vi "IMAQ Gerchberg Saxton.vi"(0 "Source":T1, 1 "Target":T1, 2 "Source Phase":T1, 3 "Target Phase":T1, 4 "n_grid":i32=300, 5 "Number of Iteration":i32=50, 6 "size_grid":dbl=0.001776, 7 "forward distance":dbl=0.02, 8 "MF Phase Refnum":refnum<vi>, 9 "FF Refnum":refnum<vi>, 10 "MF Refnum":refnum<vi>, 11 "FF Phase Refnum":refnum<vi>, 12 "lambda":dbl=1.054e-06, 13 "Target Int RMS":refnum<vi>) -> (14 "Source Intensity":dbl[][](array[numeric]), 15 "Source Phase":dbl[][](array[numeric]))   [LabVIEW 2012, in "LightPipes.lvlib"]
uses:
  LightPipes.lvlib
  <vilib>/vision/Image Controls.llb/IMAQ Image.ctl
panel:
  out "Source Phase":T1(plugin-control)
  out "Source":T1(plugin-control)
  out "Target Phase":T1(plugin-control)
  out "Target":T1(plugin-control)
  out "Iteration":i32=29
  out "Target Intensity\n RMS Error":dbl(graph)=285.2404780234725
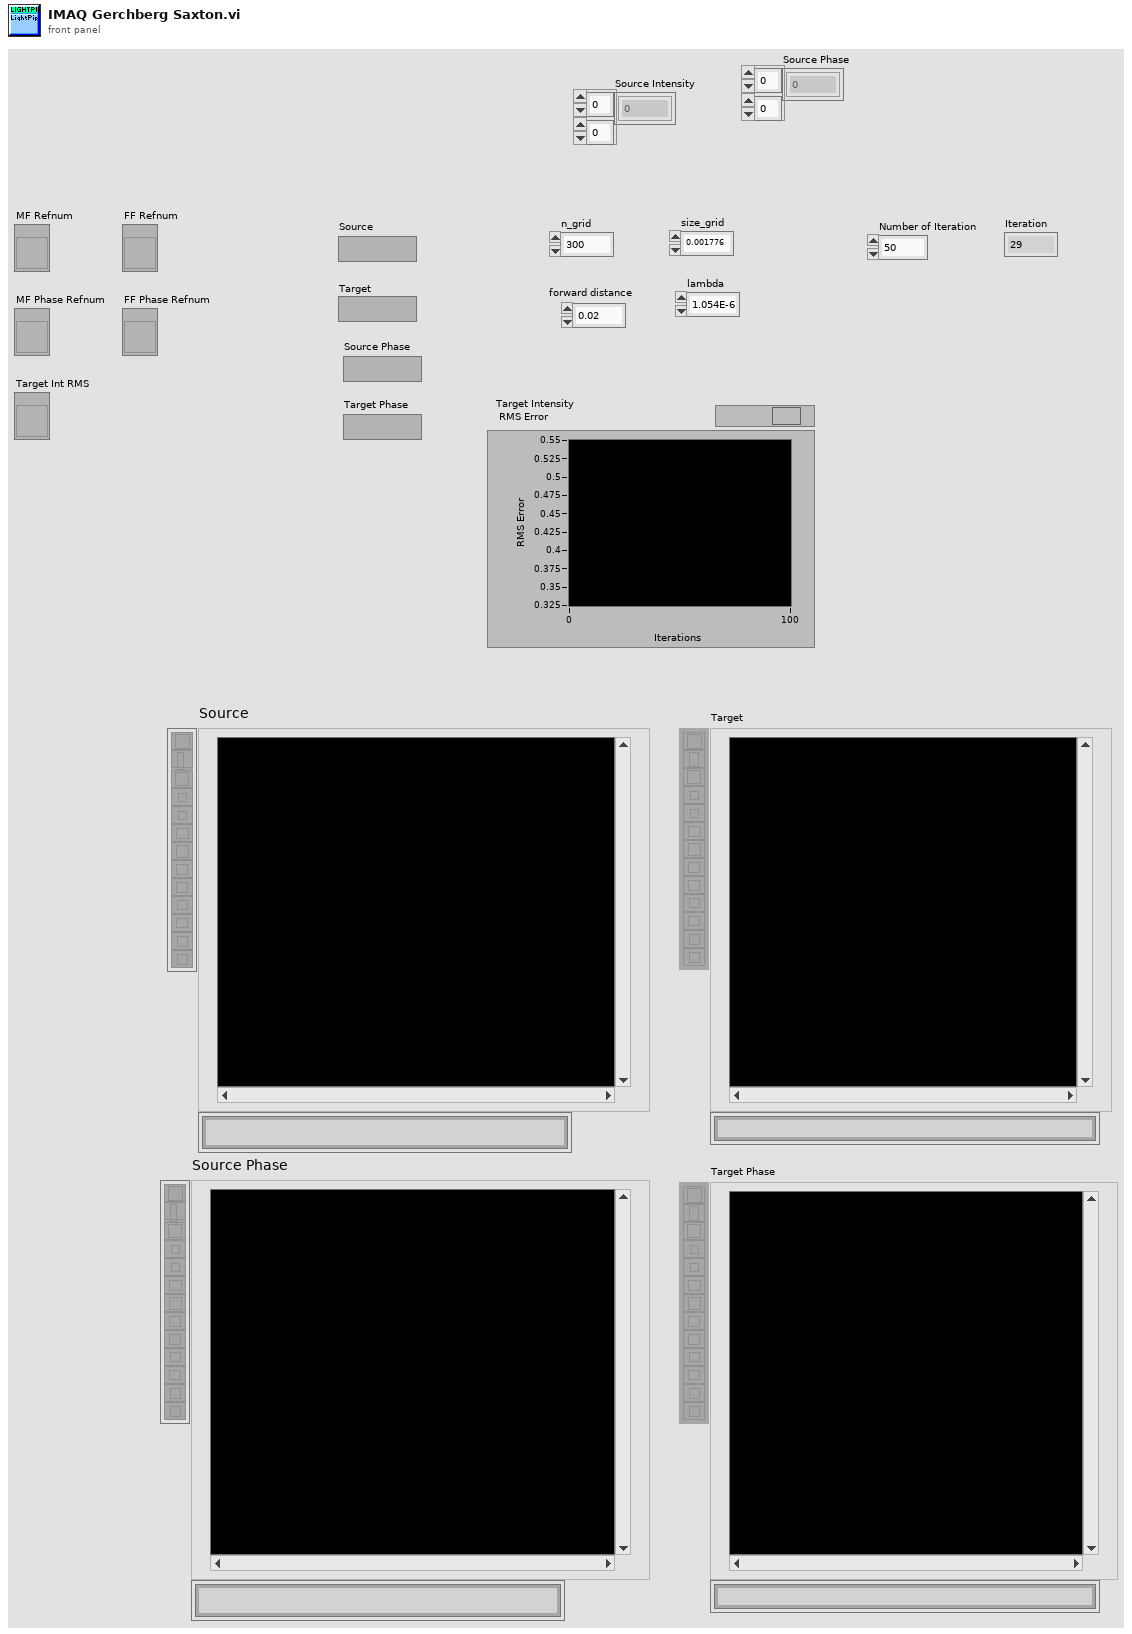
[diagram p1: front panel]
types:
  T1 = typedef "IMAQ Image.ctl" = refnum<image>
  T2 = typedef "Image Type" = u32
  T3 = cluster{"n_grid":i32, "@dummy control@":i8, "@dummy control@":i8, "@dummy control@":i8, "@dummy control@":i8, "size":dbl, "lambda":dbl, "int1":i32, "int2":i32, "int3":i32, "@dummy control@":i8, "@dummy control@":i8, "@dummy control@":i8, "@dummy control@":i8, "double1":dbl, "double2":dbl, "double3":dbl, "real":u32, "imaginary":u32}
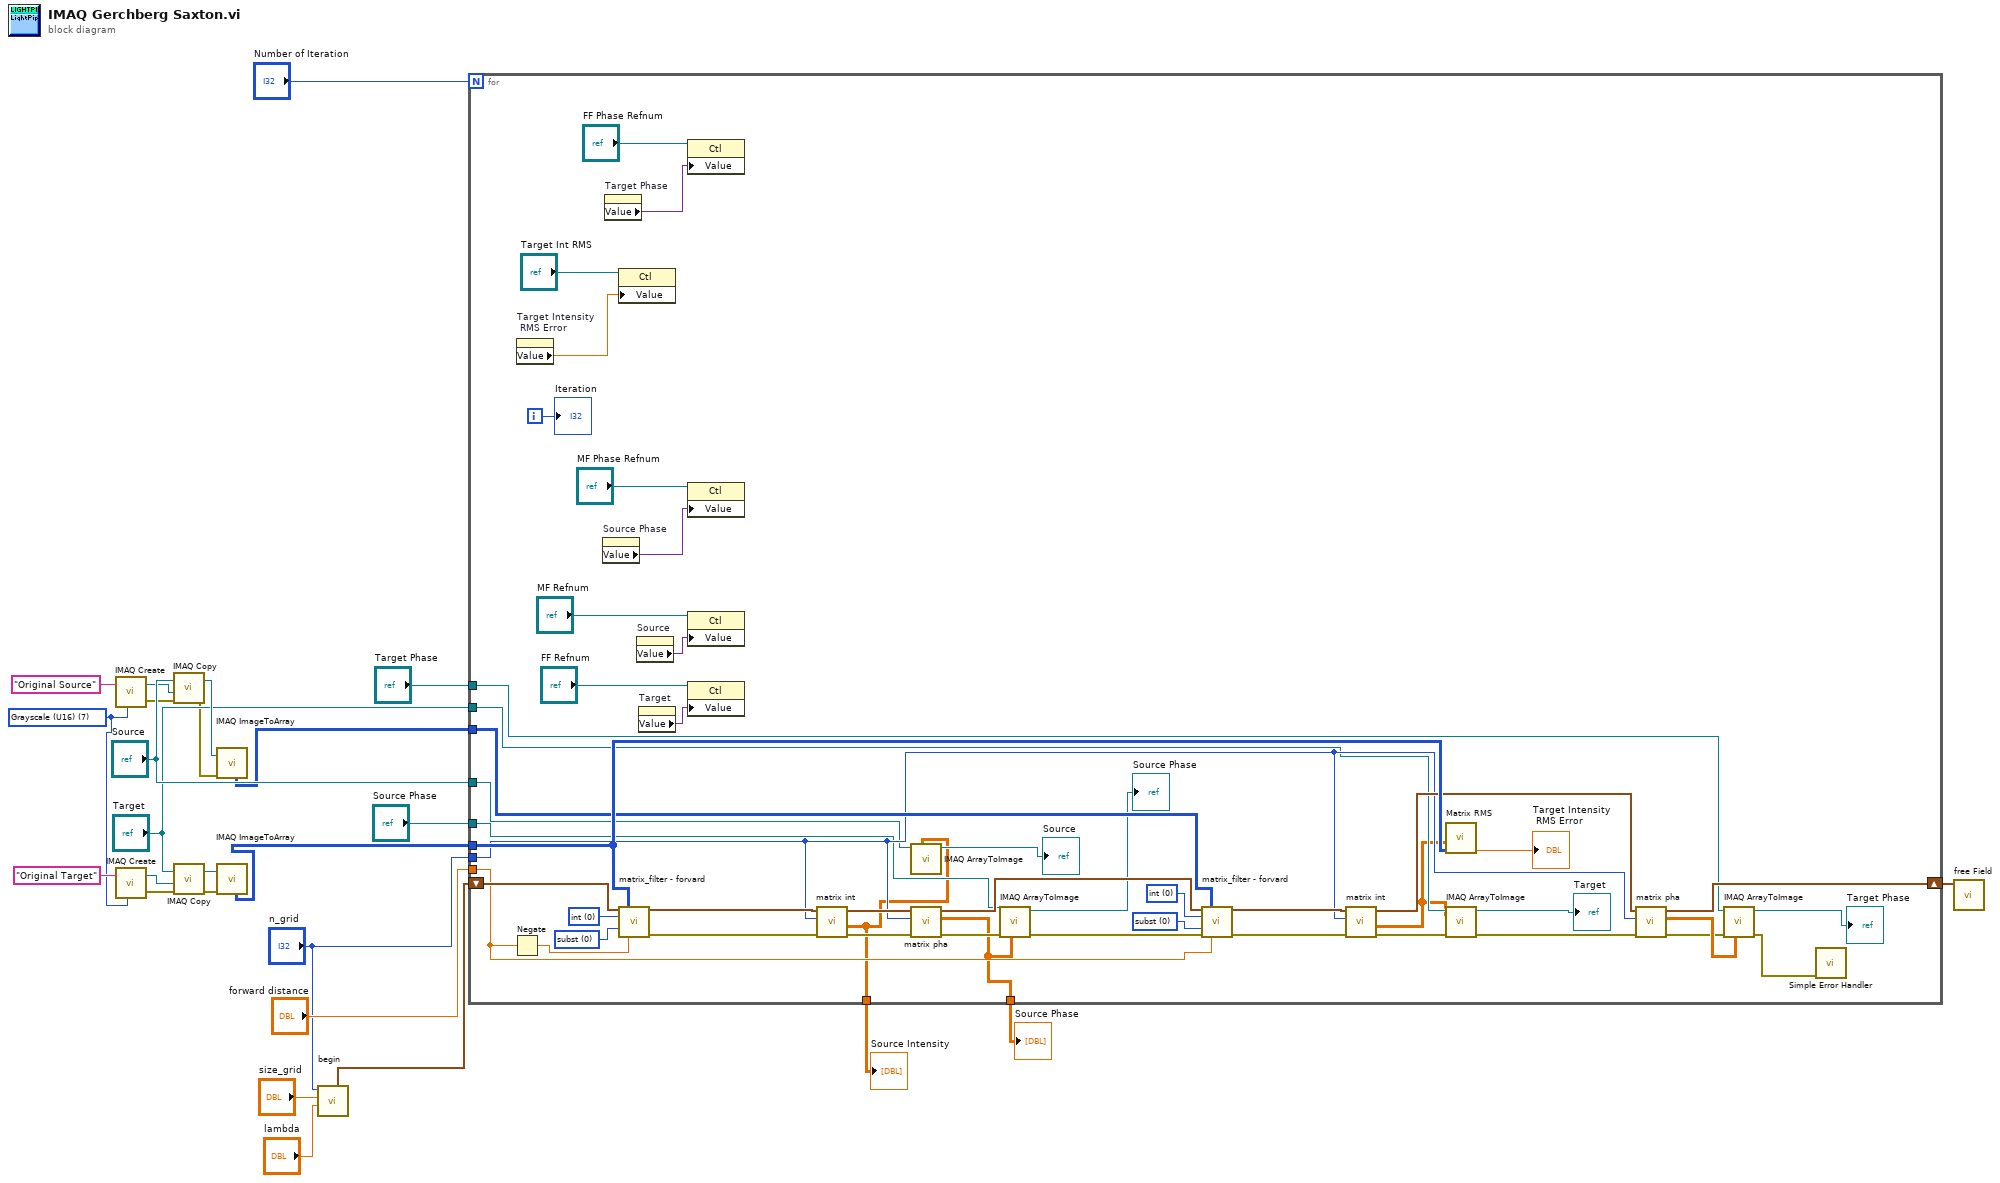
[diagram p0: block diagram]
diagram:
  w5 = T2 7 items=["Grayscale (U8)", "Grayscale (I16)", "Grayscale (SGL)", "Complex (CSG)", "RGB (U32)", "HSL (U32)", "RGB (U64)", "Grayscale (U16)"] ("Image Type")
  n1 = call "IMAQ Create"("Image Name"="Original Source", "Image Type"=w5) -> ("New Image"=w16:T1, "error out"=w15:errorcluster)  [unwired: 3 in]
  n2 = call "IMAQ Create"("Image Name"="Original Target", "Image Type"=w5) -> ("New Image"=w12:T1, "error out"=w11:errorcluster)  [unwired: 3 in]
  n3 = call "IMAQ Copy"("error in (no error)"=w15, "Image Dst"=w16, "Image Src"="Source") -> ("error out"=w7:errorcluster, "Image Dst Out"=w13:T1)  [unwired: 3 in]
  n4 = call "IMAQ Copy"("error in (no error)"=w11, "Image Dst"=w12, "Image Src"="Target") -> ("error out"=w6:errorcluster, "Image Dst Out"=w8:T1)  [unwired: 3 in]
  n5 = call "IMAQ ImageToArray"("error in (no error)"=w7, "Image"=w13) -> ("Image Pixels (U16)"=w4:u16[][])  [unwired: 2 in, 4 out]
  n6 = call "IMAQ ImageToArray"("error in (no error)"=w6, "Image"=w8) -> ("Image Pixels (U16)"=w3:u16[][])  [unwired: 2 in, 4 out]
  n7 = call "begin.vi"("lambda"="lambda", "size_grid"="size_grid", "n_grid"="n_grid") -> ("field out"=w22:T3)  [unwired: 8 in]
  n8 = for {
    N: "Number of Iteration" -> [_]
    shift-right: [w65] -> w20
    shift-left: w22 -> [w71]
    tunnel: "forward distance" -> [w39]
    tunnel: "n_grid" -> [w60]
    tunnel: w3 -> [w68]
    tunnel: w4 -> [w67]
    tunnel: "Target Phase" -> [w56]
    tunnel: "Source" -> [w55]
    tunnel: "Target" -> [w54]
    tunnel: "Source Phase" -> [w51]
    tunnel: [w28] -> w2
    tunnel: [w27] -> w1
    i -> [w66]
    w72 = i16 0 items=["int", "pha"] ("intensity/phase")
    w73 = i16 0 items=["subst", "mult"] ("multiplication/substitution")
    w74 = i16 0 items=["int", "pha"] ("intensity/phase")
    w75 = i16 0 items=["subst", "mult"] ("multiplication/substitution")
    n9 = Negate(x=w39) -> (-x=w70:dbl)
    n10 = property on="Target Intensity\n RMS Error" class="WFChart (strict)"() -> ("Value"=w44:dbl)  [unwired: 2 in, 2 out]
    n11 = property on="Source Phase" class="ImageControl"() -> ("Value"=w48:variant)  [unwired: 2 in, 2 out]
    n12 = property on="Target Phase" class="ImageControl"() -> ("Value"=w46:variant)  [unwired: 2 in, 2 out]
    n13 = property class="Ctl"(reference="Target Int RMS", "Value"=w44) -> ()  [unwired: 1 in, 2 out]
    n14 = call "matrix_filter - forvard.vi"("field"=w71, "matrix in"=w68, "intensity/phase"=w72, "multiplication/substitution"=w73, "forward distance"=w70) -> ("field out"=w63:T3, "error out"=w35:errorcluster)  [unwired: 9 in]
    n15 = property on="Source" class="ImageControl"() -> ("Value"=w42:variant)  [unwired: 2 in, 2 out]
    n16 = property on="Target" class="ImageControl"() -> ("Value"=w52:variant)  [unwired: 2 in, 2 out]
    n17 = property class="Ctl"(reference="FF Phase Refnum", "Value"=w46) -> ()  [unwired: 1 in, 2 out]
    n18 = property class="Ctl"(reference="MF Phase Refnum", "Value"=w48) -> ()  [unwired: 1 in, 2 out]
    n19 = property class="Ctl"(reference="MF Refnum", "Value"=w42) -> ()  [unwired: 1 in, 2 out]
    n20 = property class="Ctl"(reference="FF Refnum", "Value"=w52) -> ()  [unwired: 1 in, 2 out]
    n21 = call "matrix int.vi"("error in (no error)"=w35, "n_grid"=w60, "field"=w63) -> ("error out"=w36:errorcluster, "matrix out 2D"=w28:dbl[][], "field out"=w62:T3)  [unwired: 6 in]
    n22 = call "IMAQ ArrayToImage"("Image Pixels (U16)"=w28, "Image"=w55) -> ("Image Out"=→"Source":T1)  [unwired: 8 in, 1 out]
    n23 = call "matrix pha.vi"("error in (no error)"=w36, "n_grid"=w60, "field"=w62) -> ("error out"=w37:errorcluster, "matrix out 2D"=w27:dbl[][], "field out"=w61:T3)  [unwired: 6 in]
    n24 = call "IMAQ ArrayToImage"("Image Pixels (Float)"=w27, "error in (no error)"=w37, "Image"=w51) -> ("error out"=w38:errorcluster, "Image Out"=→"Source Phase":T1)  [unwired: 7 in]
    n25 = call "matrix_filter - forvard.vi"("field"=w61, "matrix in"=w67, "intensity/phase"=w74, "multiplication/substitution"=w75, "error in (no error)"=w38, "forward distance"=w39) -> ("field out"=w69:T3, "error out"=w34:errorcluster)  [unwired: 8 in]
    n26 = call "matrix int.vi"("error in (no error)"=w34, "n_grid"=w60, "field"=w69) -> ("error out"=w32:errorcluster, "matrix out 2D"=w29:dbl[][], "field out"=w64:T3)  [unwired: 6 in]
    n27 = call "Matrix RMS.vi"("Original Matrix"=w68, "Iterative Matrix"=w29) -> ("RMS"=→"Target Intensity\n RMS Error":dbl)  [unwired: 8 in, 1 out]
    n28 = call "IMAQ ArrayToImage"("Image Pixels (U16)"=w29, "error in (no error)"=w32, "Image"=w54) -> ("error out"=w31:errorcluster, "Image Out"=→"Target":T1)  [unwired: 7 in]
    n29 = call "matrix pha.vi"("error in (no error)"=w31, "n_grid"=w60, "field"=w64) -> ("error out"=w33:errorcluster, "matrix out 2D"=w40:dbl[][], "field out"=w65:T3)  [unwired: 6 in]
    n30 = call "IMAQ ArrayToImage"("Image Pixels (Float)"=w40, "error in (no error)"=w33, "Image"=w56) -> ("error out"=w30:errorcluster, "Image Out"=→"Target Phase":T1)  [unwired: 7 in]
    n31 = call <vilib>:"Simple Error Handler.vi"("error in (no error)"=w30) -> ()  [unwired: 4 in, 5 out]
    "Iteration" <- w66
  }
  "Source Intensity" <- w2
  "Source Phase" <- w1
  n32 = call "free Field.vi"("field"=w20) -> ()  [unwired: 10 in, 1 out]
